vi "mp285.vi"() -> ()   [LabVIEW 2018]
uses:
  <vilib>/Instr/_visa.llb/VISA Configure Serial Port (Instr).vi
panel:
  out "Z.":dbl
  out "Y.":dbl
  out "X.":dbl
  in  "获取当前位置":bool
  out "字符串":string
  in  "VISA资源名称":refnum<visa-resource-name>
  in  "设置精度和速度":bool
  in  "获取当前速度和位置":bool
  in  "相对运动":bool
  in  "绝对运动":bool
  in  "重置":bool
  in  "中断移动":bool
  in  "设置当前位置为原点":bool
  in  "停止":bool
  out "速度":dbl
  out "精度":u16
  in  "速度":dbl
  in  "精度":u16(ring)=10 items=["Low (10microsteps/step)", "High (50microsteps/step)"]
  out "错误输出":errorcluster
  in  "Abso_Z":dbl
  in  "Abso_Y":dbl
  in  "Abso_X":dbl
  in  "Z":dbl
  in  "Y":dbl
  in  "X":dbl
  in  "停止位 (10: 1位)":u16(ring)=10 caption="停止位(1)" items=["1.0"=10, "1.5"=15, "2.0"=20]
  in  "校验（无）":enum16{"None", "Odd", "Even", "Mark", "Space"}(ring)
  in  "波特率(9600)":u32=9600
  # "当前位置\n（单位：微米）"
  # "移动到绝对位置\n（单位：微米）"
  # "移动到相对位置\n（单位：微米）"
  # "串口设置"
  # "获取精度和速度"
  # "设置精度和速度"
  # "速度范围：低精度模式下0-3000微米/秒\n               高精度模式下0-1310微米/秒"
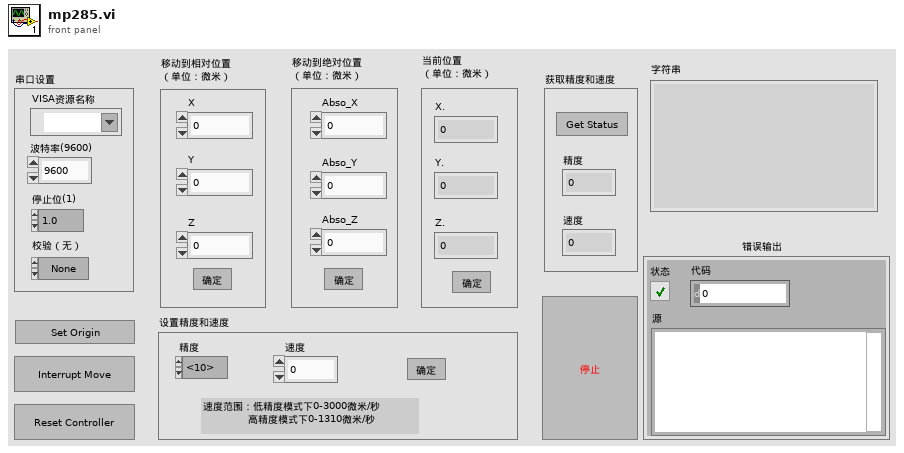
[diagram p1: front panel]
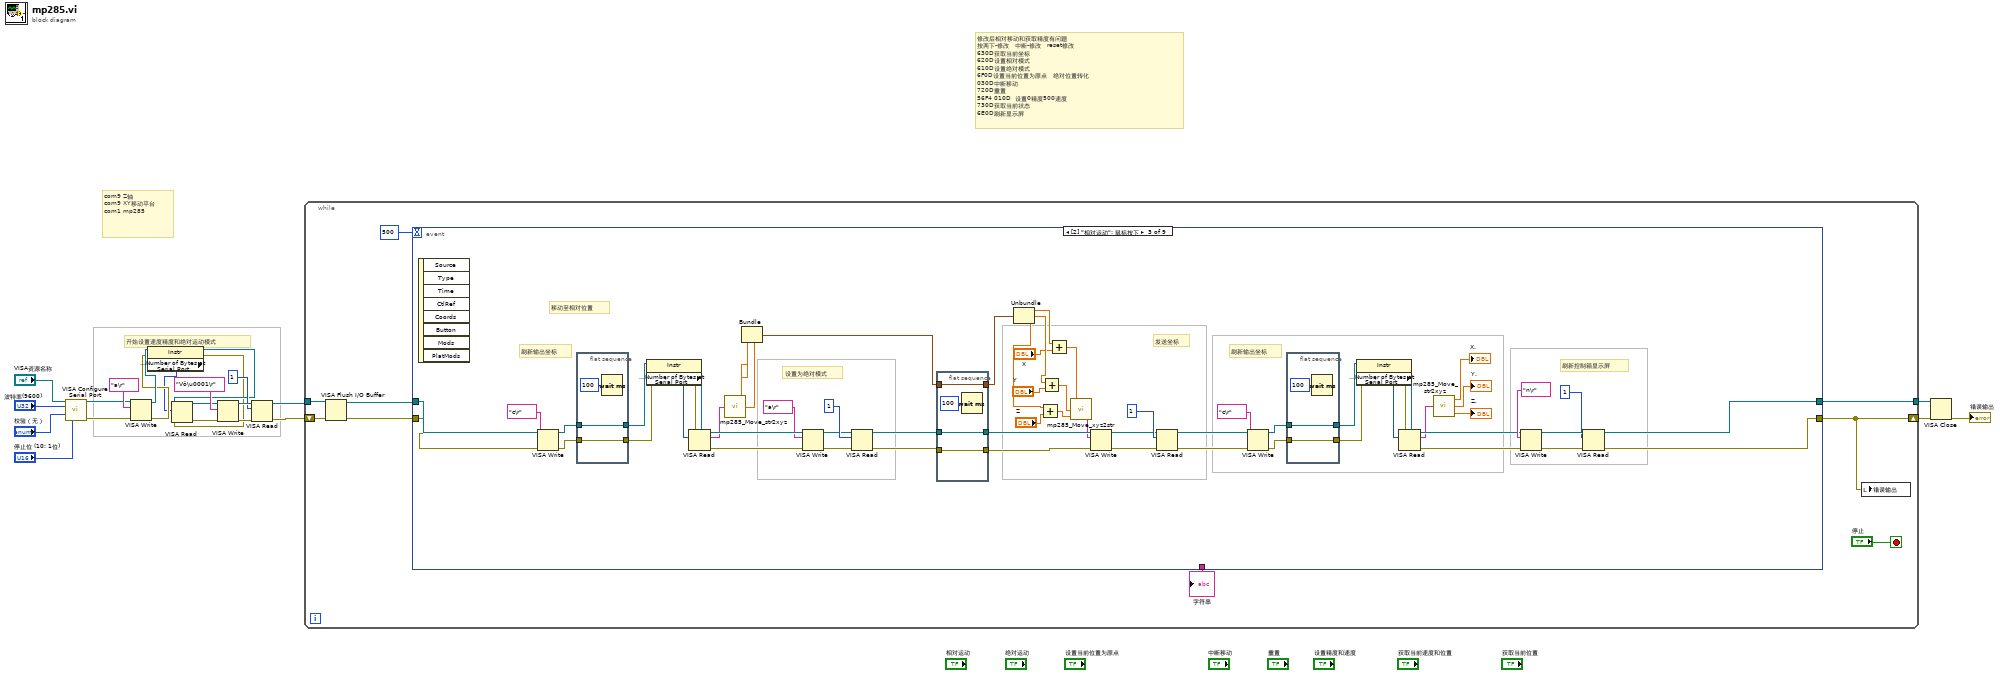
[diagram p0: block diagram]
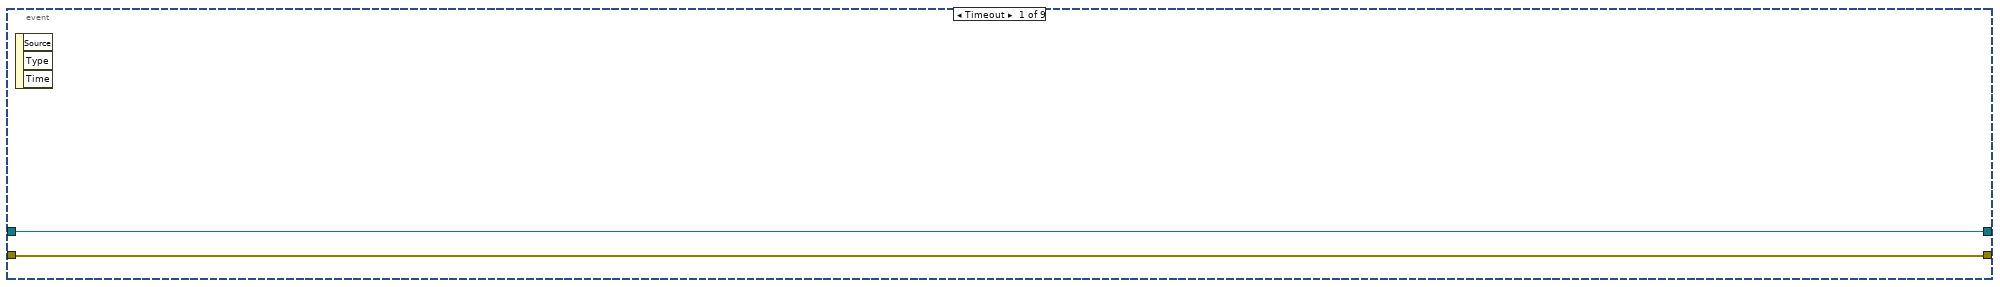
[diagram p2: hidden frame]
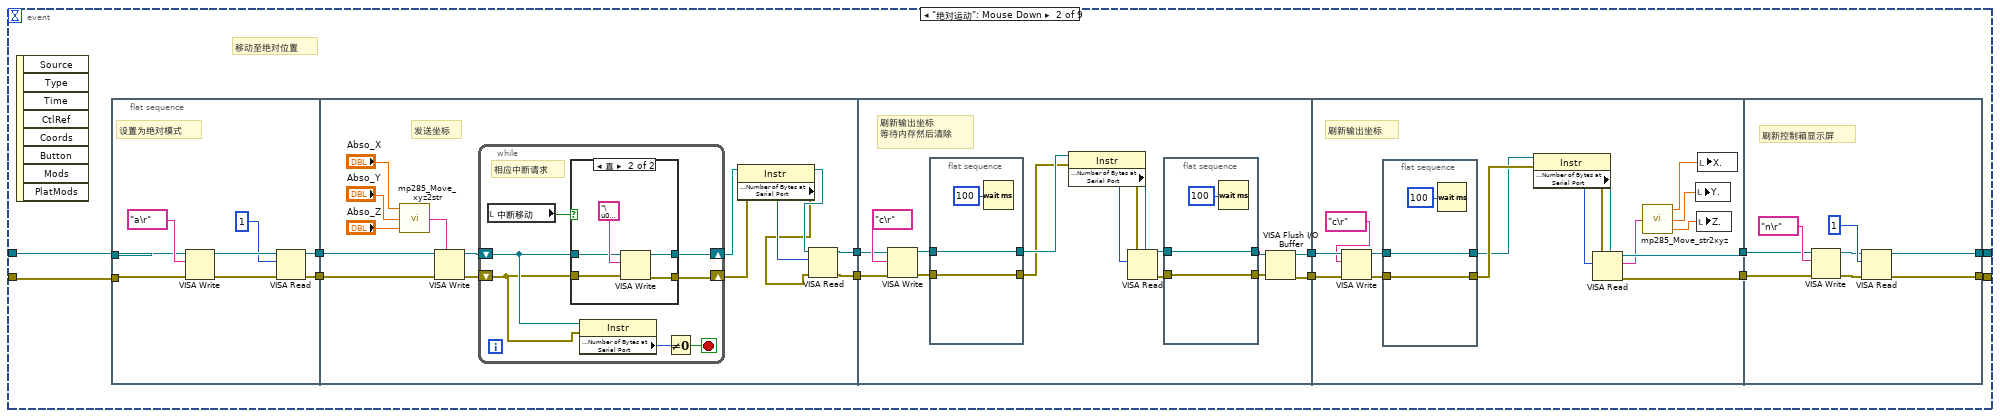
[diagram p3: hidden frame]
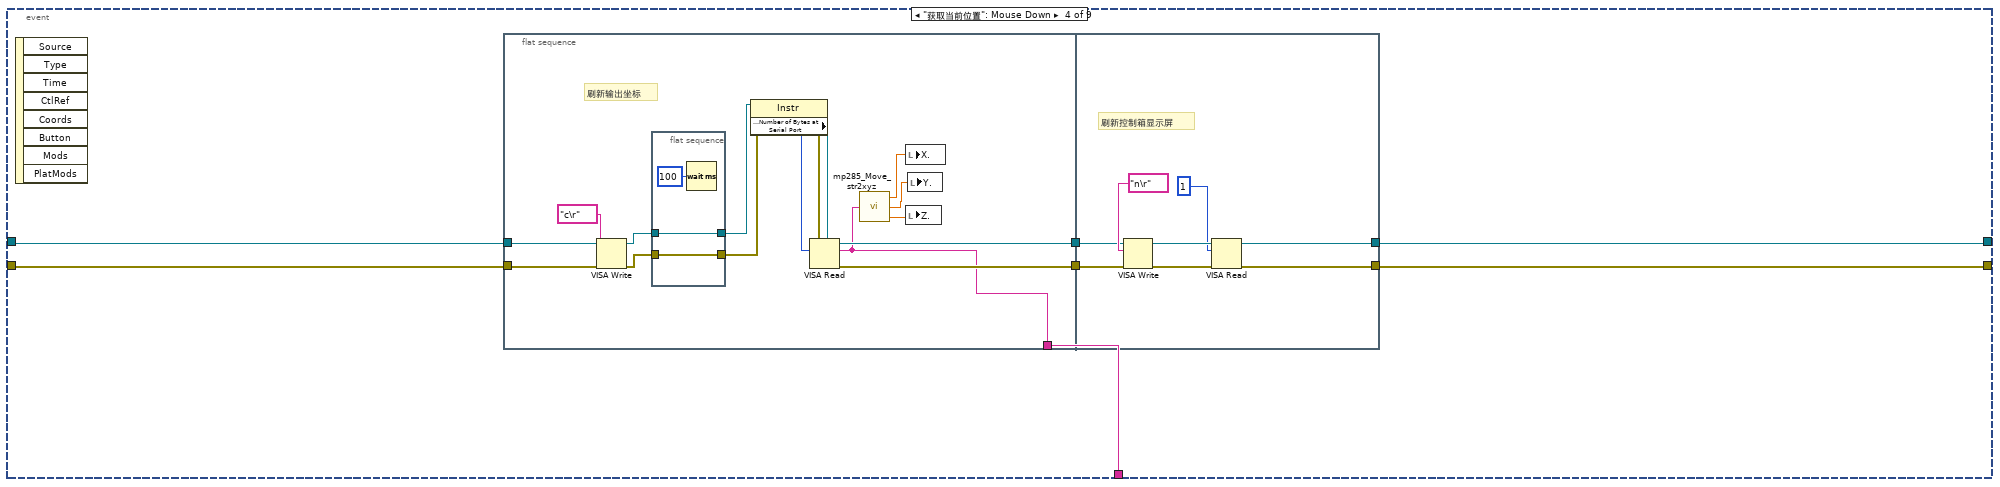
[diagram p5: hidden frame]
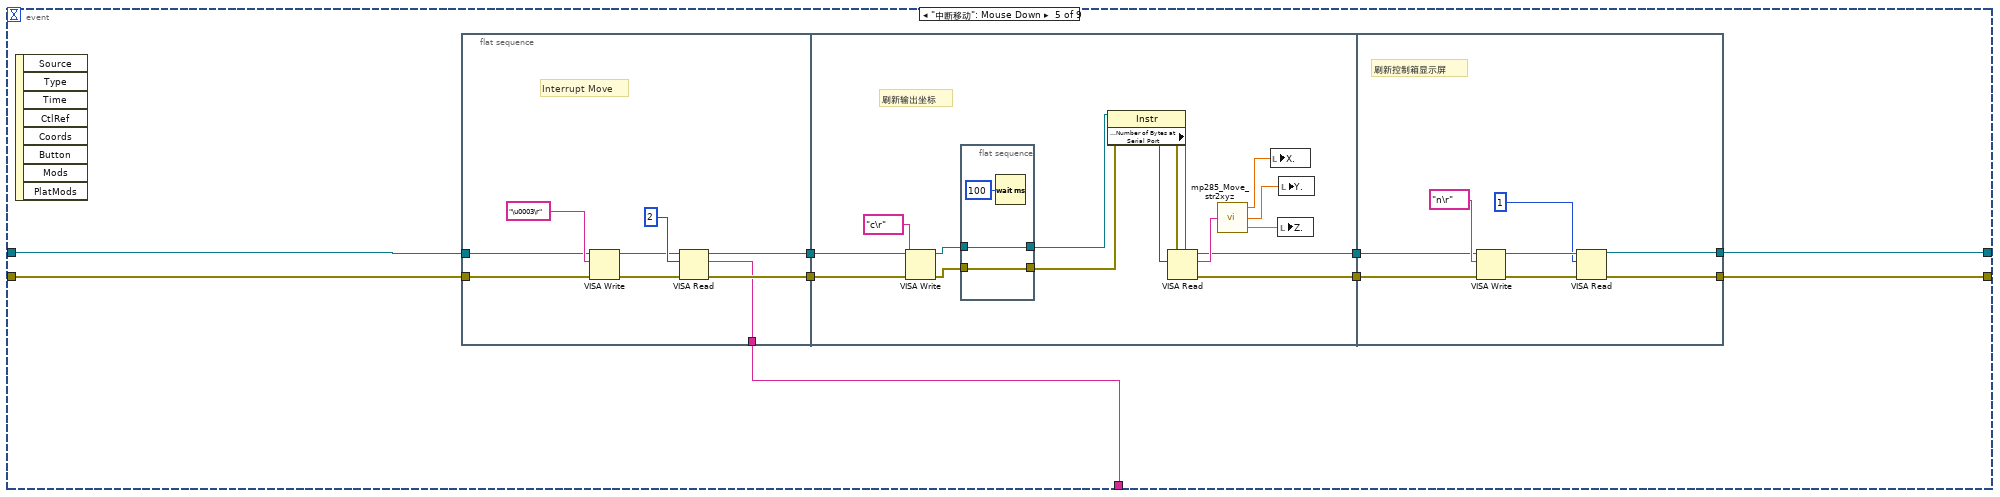
[diagram p6: hidden frame]
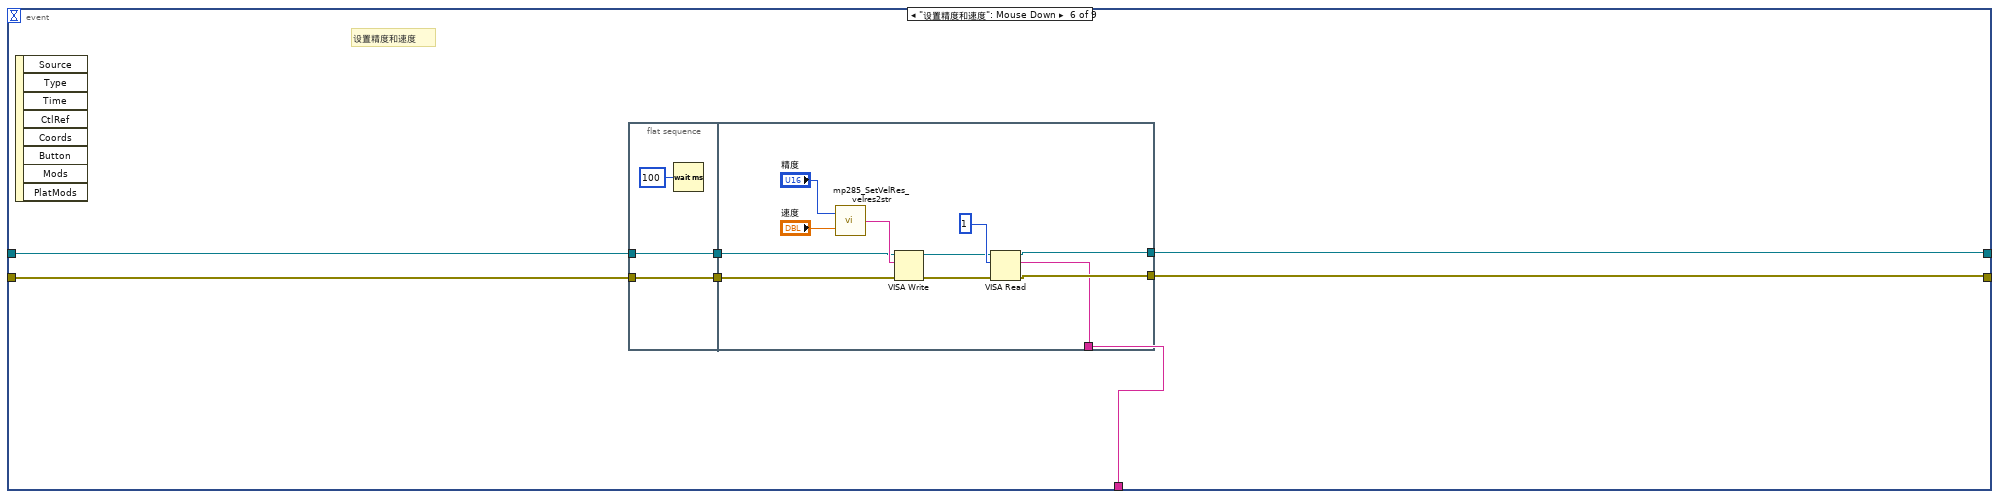
[diagram p7: hidden frame]
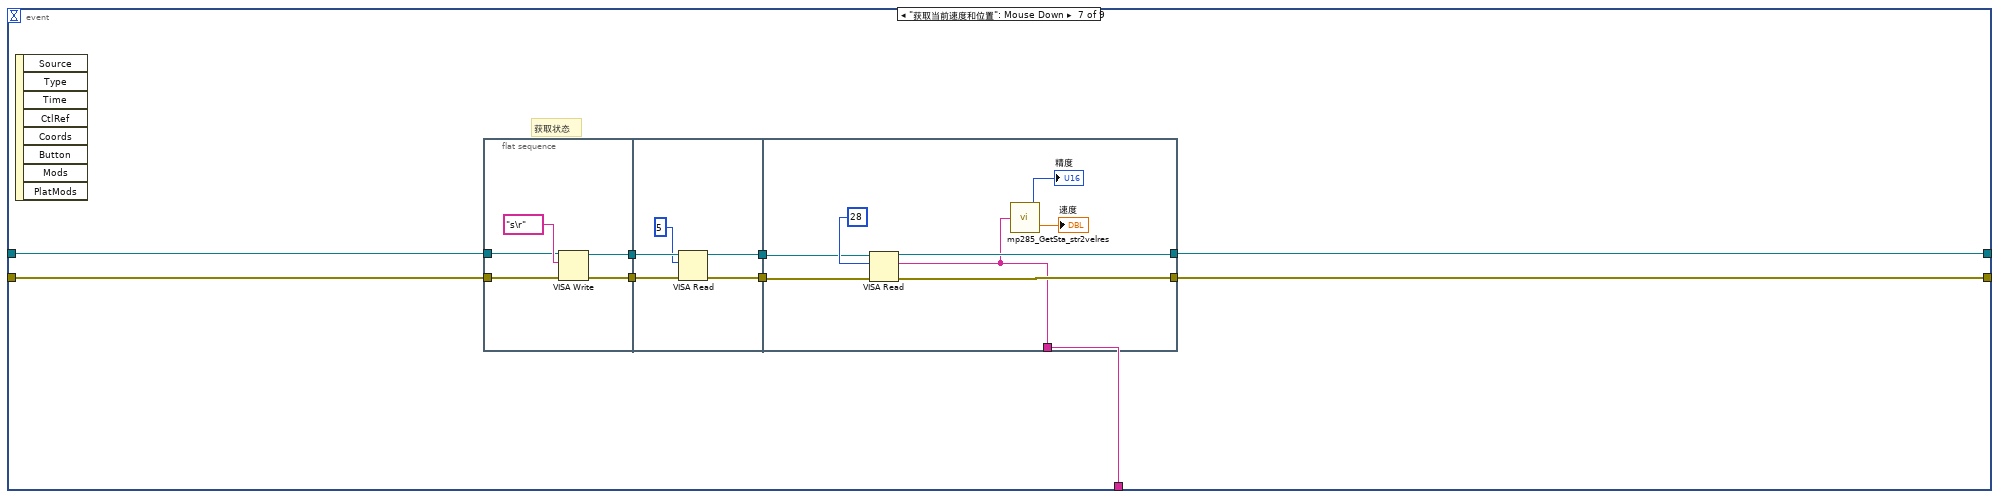
[diagram p8: hidden frame]
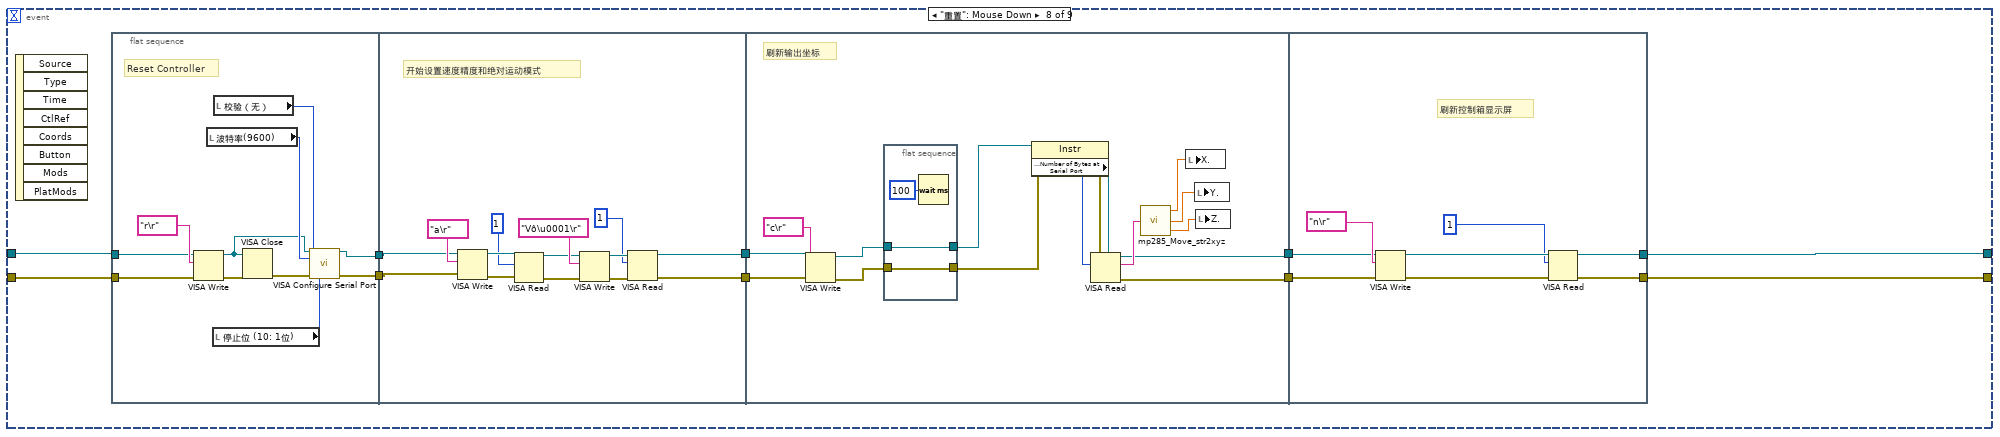
[diagram p9: hidden frame]
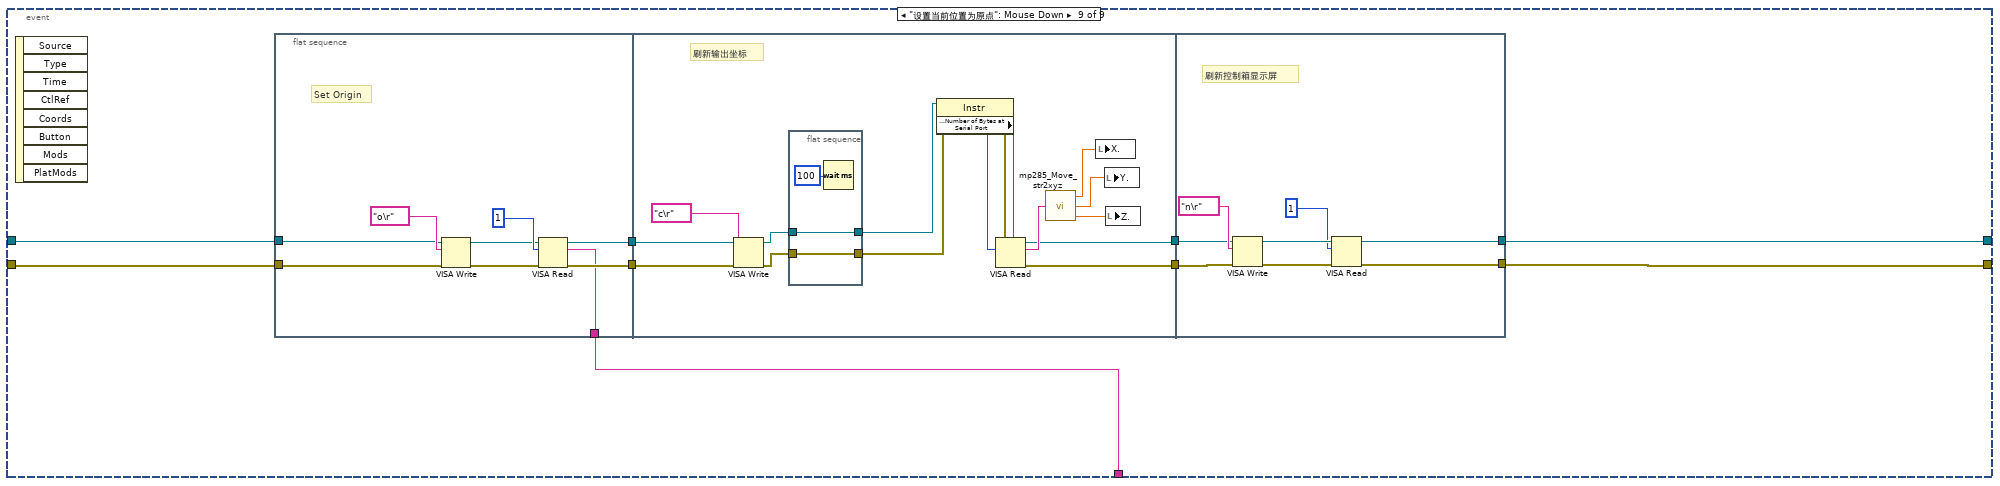
[diagram p10: hidden frame]
diagram:
  # "com9 Z轴\ncom9 XY移动平台\ncom1 mp285"
  # "开始设置速度精度和绝对运动模式"
  # "修改后相对移动和获取精度有问题\n按两下-修改   中断-修改   reset修改\n630D获取当前坐标\n620D设置相对模式\n610D设置绝对模式\n6F0D设置当前位置为原点   绝对位置转化\n030D中断移动\n720D重置\n56F4 010D  设置0精度500速度\n730D获取当前状态\n6E0D刷新显示屏"
  n1 = call-poly "VISA Configure Serial Port"("VISA resource name"="VISA资源名称", "baud rate (9600)"="波特率(9600)", "parity (0:none)"="校验（无）", "stop bits (10: 1 bit)"="停止位 (10: 1位)") -> ("VISA resource name out"=w7:refnum<visa-resource-name>, "error out"=w6:errorcluster)  [unwired: 10 in]
  n2 = VISA Write ("VISA写入")(VISA resource name=w7, write buffer="a\r" ("写入缓冲区"), error in (no error)=w6) -> (VISA resource name out=w5:refnum<visa-resource-name>, error out=w4:errorcluster)  [unwired: 1 out]
  n3 = property class="Instr"(reference=w5, error in=w4) -> (reference out=w3:refnum<visa-resource-name>, error out=w1:errorcluster, "Serial Settings:Number of Bytes at Serial Port"=w2:u32)
  n4 = VISA Read(VISA resource name=w3, byte count=w2, error in (no error)=w1) -> (VISA resource name out=w14:refnum<visa-resource-name>, error out=w13:errorcluster)  [unwired: 2 out]
  n5 = VISA Write ("VISA写入")(VISA resource name=w14, write buffer="Vô\u0001\r" ("写入缓冲区"), error in (no error)=w13) -> (VISA resource name out=w11:refnum<visa-resource-name>, error out=w12:errorcluster)  [unwired: 1 out]
  n6 = VISA Read(VISA resource name=w11, byte count=u32 1 ("字节总数"), error in (no error)=w12) -> (VISA resource name out=w10:refnum<visa-resource-name>, error out=w8:errorcluster)  [unwired: 2 out]
  n7 = while {
    tunnel: w10 -> [w27]
    tunnel: [w31] -> w18
    shift-right: [w28] -> w17
    shift-left: w8 -> [w25]
    stop <- "停止" stop-if-true
    n8 = VISA Flush I/O Buffer(VISA resource name=w27, error in (no error)=w25) -> (VISA resource name out=w26:refnum<visa-resource-name>, error out=w24:errorcluster)  [unwired: 1 in]
    n9 = event shown="[2] \"相对运动\": 鼠标按下" {
      selector: _ -> [_ _ _ _ _ _ _ _ _]
      dyn-events: _ -> [_ _ _ _ _ _ _ _ _]
      timeout: 500 -> [_ _ _ _ _ _ _ _ _]
      tunnel: w26 -> [w34 w46 w143 w210 w245 w289 w305 w340 w401]
      tunnel: w24 -> [w33 w45 w142 w209 w246 w288 w304 w339 w400]
      tunnel: [w33 w39 w137 w204 w238 w286 w307 w331 w393] -> w28
      tunnel: [w34 w40 w138 w205 w239 w287 w308 w332 w394] -> w31
      tunnel: [_ _ _ w208 w244 w285 w306 _ w399] -> w30
      event Timeout {
        n10 = event-data() -> ()  [unwired: 1 in, 3 out]
      }
      event "绝对运动": Mouse Down {
        # "移动至绝对位置"
        n11 = event-data() -> ()  [unwired: 1 in, 8 out]
        n12 = flat-sequence {
          tunnel: w46 -> [w50]
          tunnel: w45 -> [w49]
          tunnel: [w48] -> w44
          tunnel: [w47] -> w43
          tunnel: w44 -> [w59]
          tunnel: w43 -> [w58]
          tunnel: [w57] -> w42
          tunnel: [w56] -> w41
          tunnel: w42 -> [w95]
          tunnel: w41 -> [w94]
          tunnel: [w88] -> w38
          tunnel: [w89] -> w37
          tunnel: w38 -> [w114]
          tunnel: w37 -> [w113]
          tunnel: [w111] -> w36
          tunnel: [w110] -> w35
          tunnel: [w129] -> w40
          tunnel: [w128] -> w39
          tunnel: w36 -> [w126]
          tunnel: w35 -> [w125]
          frame #0 {
            # "设置为绝对模式"
            n13 = VISA Write ("VISA写入")(VISA resource name=w50, write buffer="a\r" ("写入缓冲区"), error in (no error)=w49) -> (VISA resource name out=w53:refnum<visa-resource-name>, error out=w52:errorcluster)  [unwired: 1 out]
            n14 = VISA Read(VISA resource name=w53, byte count=u32 1 ("字节总数"), error in (no error)=w52) -> (VISA resource name out=w47:refnum<visa-resource-name>, error out=w48:errorcluster)  [unwired: 2 out]
          }
          frame #1 {
            # "发送坐标"
            n15 = call "mp285_Move_xyz2str.vi"("Z轴"="Abso_Z", "Y轴"="Abso_Y", "X轴"="Abso_X") -> ("发送至串口的字符串"=w69:string)
            n16 = VISA Write ("VISA写入")(VISA resource name=w58, write buffer=w69, error in (no error)=w59) -> (VISA resource name out=w65:refnum<visa-resource-name>, error out=w64:errorcluster)  [unwired: 1 out]
            n17 = while {
              shift-right: [w75] -> w63
              shift-left: w65 -> [w73]
              shift-right: [w74] -> w62
              shift-left: w64 -> [w72]
              stop <- w71 stop-if-true
              # "相应中断请求"
              n18 = local read "中断移动"() -> (w76:bool)
              n19 = case shown="真" w76 {
                tunnel: [w77 w80] -> w75
                tunnel: [w78 w79] -> w74
                tunnel: w73 -> [w77 w82]
                tunnel: w72 -> [w78 w81]
                frame False {
                }
                frame True {
                  n20 = VISA Write ("VISA写入")(VISA resource name=w82, write buffer="\u0003" ("写入缓冲区"), error in (no error)=w81) -> (VISA resource name out=w80:refnum<visa-resource-name>, error out=w79:errorcluster)  [unwired: 1 out]
                }
              }
              n21 = property class="Instr"(reference=w73, error in=w72) -> ("Serial Settings:Number of Bytes at Serial Port"=w70:u32)  [unwired: 2 out]
              n22 = Not Equal To 0?(x=w70) -> (x != 0?=w71:bool)
            }
            n23 = property class="Instr"(reference=w63, error in=w62) -> (reference out=w61:refnum<visa-resource-name>, error out=w55:errorcluster, "Serial Settings:Number of Bytes at Serial Port"=w60:u32)
            n24 = VISA Read(VISA resource name=w61, byte count=w60, error in (no error)=w55) -> (VISA resource name out=w57:refnum<visa-resource-name>, error out=w56:errorcluster)  [unwired: 2 out]
          }
          frame #2 {
            # "刷新输出坐标\n等待内存然后清除"
            n25 = VISA Write ("VISA写入")(VISA resource name=w95, write buffer="c\r" ("写入缓冲区"), error in (no error)=w94) -> (VISA resource name out=w93:refnum<visa-resource-name>, error out=w92:errorcluster)  [unwired: 1 out]
            n26 = flat-sequence {
              tunnel: w93 -> [w104]
              tunnel: w92 -> [w103]
              tunnel: [w104] -> w91
              tunnel: [w103] -> w90
              frame #0 {
                n27 = Wait (ms)(milliseconds to wait=u32 100 ("等待时间（毫秒）")) -> ()  [unwired: 1 out]
              }
            }
            n28 = property class="Instr"(reference=w91, error in=w90) -> (reference out=w98:refnum<visa-resource-name>, error out=w99:errorcluster, "Serial Settings:Number of Bytes at Serial Port"=w97:u32)
            n29 = VISA Read(VISA resource name=w98, byte count=w97, error in (no error)=w99) -> (VISA resource name out=w87:refnum<visa-resource-name>, error out=w86:errorcluster)  [unwired: 2 out]
            n30 = flat-sequence {
              tunnel: w87 -> [w101]
              tunnel: w86 -> [w100]
              tunnel: [w101] -> w85
              tunnel: [w100] -> w84
              frame #0 {
                n31 = Wait (ms)(milliseconds to wait=u32 100 ("等待时间（毫秒）")) -> ()  [unwired: 1 out]
              }
            }
            n32 = VISA Flush I/O Buffer(VISA resource name=w85, error in (no error)=w84) -> (VISA resource name out=w88:refnum<visa-resource-name>, error out=w89:errorcluster)  [unwired: 1 in]
          }
          frame #3 {
            # "刷新输出坐标"
            n33 = VISA Write ("VISA写入")(VISA resource name=w114, write buffer="c\r" ("写入缓冲区"), error in (no error)=w113) -> (VISA resource name out=w118:refnum<visa-resource-name>, error out=w119:errorcluster)  [unwired: 1 out]
            n34 = flat-sequence {
              tunnel: w118 -> [w123]
              tunnel: w119 -> [w122]
              tunnel: [w123] -> w120
              tunnel: [w122] -> w121
              frame #0 {
                n35 = Wait (ms)(milliseconds to wait=u32 100 ("等待时间（毫秒）")) -> ()  [unwired: 1 out]
              }
            }
            n36 = property class="Instr"(reference=w120, error in=w121) -> (reference out=w116:refnum<visa-resource-name>, error out=w115:errorcluster, "Serial Settings:Number of Bytes at Serial Port"=w117:u32)
            n37 = VISA Read(VISA resource name=w116, byte count=w117, error in (no error)=w115) -> (VISA resource name out=w111:refnum<visa-resource-name>, read buffer=w109:string, error out=w110:errorcluster)  [unwired: 1 out]
            n38 = call "mp285_Move_str2xyz.vi"("字符串"=w109) -> ("X轴"=w108:dbl, "Y轴"=w107:dbl, "Z轴"=w106:dbl)
            n39 = local write "Y."(w107) -> ()
            n40 = local write "Z."(w106) -> ()
            n41 = local write "X."(w108) -> ()
          }
          frame #4 {
            # "刷新控制箱显示屏"
            n42 = VISA Write ("VISA写入")(VISA resource name=w126, write buffer="n\r" ("写入缓冲区"), error in (no error)=w125) -> (VISA resource name out=w131:refnum<visa-resource-name>, error out=w130:errorcluster)  [unwired: 1 out]
            n43 = VISA Read(VISA resource name=w131, byte count=u32 1 ("字节总数"), error in (no error)=w130) -> (VISA resource name out=w129:refnum<visa-resource-name>, error out=w128:errorcluster)  [unwired: 2 out]
          }
        }
      }
      event "相对运动": Mouse Down {
        # "刷新输出坐标"
        # "刷新输出坐标"
        # "刷新控制箱显示屏"
        # "设置为绝对模式"
        # "发送坐标"
        # "移动至相对位置"
        n44 = event-data() -> ()  [unwired: 1 in, 8 out]
        n45 = VISA Write ("VISA写入")(VISA resource name=w143, write buffer="c\r" ("写入缓冲区"), error in (no error)=w142) -> (VISA resource name out=w171:refnum<visa-resource-name>, error out=w170:errorcluster)  [unwired: 1 out]
        n46 = flat-sequence {
          tunnel: [w199] -> w168
          tunnel: w171 -> [w199]
          tunnel: [w198] -> w169
          tunnel: w170 -> [w198]
          frame #0 {
            n47 = Wait (ms)(milliseconds to wait=u32 100 ("等待时间（毫秒）")) -> ()  [unwired: 1 out]
          }
        }
        n48 = property class="Instr"(reference=w168, error in=w169) -> (reference out=w173:refnum<visa-resource-name>, error out=w172:errorcluster, "Serial Settings:Number of Bytes at Serial Port"=w174:u32)
        n49 = VISA Read(VISA resource name=w173, byte count=w174, error in (no error)=w172) -> (VISA resource name out=w180:refnum<visa-resource-name>, read buffer=w176:string, error out=w181:errorcluster)  [unwired: 1 out]
        n50 = call "mp285_Move_str2xyz.vi"("字符串"=w176) -> ("X轴"=w184:dbl, "Y轴"=w185:dbl, "Z轴"=w186:dbl)
        n51 = Bundle("X轴"=w184, "Y轴"=w185, "Z轴"=w186) -> (w189:cluster{"X轴":dbl, "Y轴":dbl, "Z轴":dbl})  [unwired: 1 in]
        n52 = VISA Write ("VISA写入")(VISA resource name=w180, write buffer="a\r" ("写入缓冲区"), error in (no error)=w181) -> (VISA resource name out=w144:refnum<visa-resource-name>, error out=w145:errorcluster)  [unwired: 1 out]
        n53 = VISA Read(VISA resource name=w144, byte count=u32 1 ("字节总数"), error in (no error)=w145) -> (VISA resource name out=w187:refnum<visa-resource-name>, error out=w188:errorcluster)  [unwired: 2 out]
        n54 = flat-sequence {
          tunnel: w187 -> [w196]
          tunnel: w188 -> [w195]
          tunnel: [w196] -> w182
          tunnel: [w195] -> w183
          tunnel: w189 -> [w194]
          tunnel: [w194] -> w190
          frame #0 {
            n55 = Wait (ms)(milliseconds to wait=u32 100 ("等待时间（毫秒）")) -> ()  [unwired: 1 out]
          }
        }
        n56 = Unbundle(w190) -> ("X轴"=w191:dbl, "Y轴"=w192:dbl, "Z轴"=w193:dbl)
        n57 = Add(x=w193, y="Z") -> (x+y=w177:dbl)
        n58 = Add(x=w192, y="Y") -> (x+y=w178:dbl)
        n59 = Add(x=w191, y="X") -> (x+y=w179:dbl)
        n60 = call "mp285_Move_xyz2str.vi"("Z轴"=w177, "Y轴"=w178, "X轴"=w179) -> ("发送至串口的字符串"=w150:string)
        n61 = VISA Write ("VISA写入")(VISA resource name=w182, write buffer=w150, error in (no error)=w183) -> (VISA resource name out=w148:refnum<visa-resource-name>, error out=w147:errorcluster)  [unwired: 1 out]
        n62 = VISA Read(VISA resource name=w148, byte count=u32 1 ("字节总数"), error in (no error)=w147) -> (VISA resource name out=w166:refnum<visa-resource-name>, error out=w167:errorcluster)  [unwired: 2 out]
        n63 = VISA Write ("VISA写入")(VISA resource name=w166, write buffer="c\r" ("写入缓冲区"), error in (no error)=w167) -> (VISA resource name out=w155:refnum<visa-resource-name>, error out=w154:errorcluster)  [unwired: 1 out]
        n64 = flat-sequence {
          tunnel: [w202] -> w152
          tunnel: w155 -> [w202]
          tunnel: [w201] -> w153
          tunnel: w154 -> [w201]
          frame #0 {
            n65 = Wait (ms)(milliseconds to wait=u32 100 ("等待时间（毫秒）")) -> ()  [unwired: 1 out]
          }
        }
        n66 = property class="Instr"(reference=w152, error in=w153) -> (reference out=w157:refnum<visa-resource-name>, error out=w156:errorcluster, "Serial Settings:Number of Bytes at Serial Port"=w158:u32)
        n67 = VISA Read(VISA resource name=w157, byte count=w158, error in (no error)=w156) -> (VISA resource name out=w160:refnum<visa-resource-name>, read buffer=w136:string, error out=w159:errorcluster)  [unwired: 1 out]
        n68 = call "mp285_Move_str2xyz.vi"("字符串"=w136) -> ("X轴"=→"X.":dbl, "Y轴"=→"Y.":dbl, "Z轴"=→"Z.":dbl)
        n69 = VISA Write ("VISA写入")(VISA resource name=w160, write buffer="n\r" ("写入缓冲区"), error in (no error)=w159) -> (VISA resource name out=w164:refnum<visa-resource-name>, error out=w165:errorcluster)  [unwired: 1 out]
        n70 = VISA Read(VISA resource name=w164, byte count=u32 1 ("字节总数"), error in (no error)=w165) -> (VISA resource name out=w138:refnum<visa-resource-name>, error out=w137:errorcluster)  [unwired: 2 out]
      }
      event "获取当前位置": Mouse Down {
        n71 = event-data() -> ()  [unwired: 1 in, 8 out]
        n72 = flat-sequence {
          tunnel: w210 -> [w216]
          tunnel: w209 -> [w215]
          tunnel: [w214] -> w208
          tunnel: [w219] -> w207
          tunnel: [w218] -> w206
          tunnel: w207 -> [w232]
          tunnel: w206 -> [w233]
          tunnel: [w231] -> w205
          tunnel: [w230] -> w204
          frame #0 {
            # "刷新输出坐标"
            n73 = VISA Write ("VISA写入")(VISA resource name=w216, write buffer="c\r" ("写入缓冲区"), error in (no error)=w215) -> (VISA resource name out=w223:refnum<visa-resource-name>, error out=w224:errorcluster)  [unwired: 1 out]
            n74 = flat-sequence {
              tunnel: [w228] -> w226
              tunnel: w223 -> [w228]
              tunnel: [w227] -> w225
              tunnel: w224 -> [w227]
              frame #0 {
                n75 = Wait (ms)(milliseconds to wait=u32 100 ("等待时间（毫秒）")) -> ()  [unwired: 1 out]
              }
            }
            n76 = property class="Instr"(reference=w226, error in=w225) -> (reference out=w221:refnum<visa-resource-name>, error out=w222:errorcluster, "Serial Settings:Number of Bytes at Serial Port"=w220:u32)
            n77 = VISA Read(VISA resource name=w221, byte count=w220, error in (no error)=w222) -> (VISA resource name out=w218:refnum<visa-resource-name>, read buffer=w214:string, error out=w219:errorcluster)  [unwired: 1 out]
            n78 = call "mp285_Move_str2xyz.vi"("字符串"=w214) -> ("X轴"=w213:dbl, "Y轴"=w212:dbl, "Z轴"=w211:dbl)
            n79 = local write "X."(w213) -> ()
            n80 = local write "Z."(w211) -> ()
            n81 = local write "Y."(w212) -> ()
          }
          frame #1 {
            # "刷新控制箱显示屏"
            n82 = VISA Write ("VISA写入")(VISA resource name=w233, write buffer="n\r" ("写入缓冲区"), error in (no error)=w232) -> (VISA resource name out=w236:refnum<visa-resource-name>, error out=w237:errorcluster)  [unwired: 1 out]
            n83 = VISA Read(VISA resource name=w236, byte count=u32 1 ("字节总数"), error in (no error)=w237) -> (VISA resource name out=w231:refnum<visa-resource-name>, error out=w230:errorcluster)  [unwired: 2 out]
          }
        }
      }
      event "中断移动": Mouse Down {
        n84 = event-data() -> ()  [unwired: 1 in, 8 out]
        n85 = flat-sequence {
          tunnel: w246 -> [w252]
          tunnel: w245 -> [w251]
          tunnel: [w247] -> w244
          tunnel: [w249] -> w243
          tunnel: [w248] -> w242
          tunnel: w243 -> [w262]
          tunnel: w242 -> [w261]
          tunnel: [w260] -> w241
          tunnel: [w259] -> w240
          tunnel: w241 -> [w278]
          tunnel: w240 -> [w277]
          tunnel: [w276] -> w239
          tunnel: [w275] -> w238
          frame #0 {
            # "Interrupt Move"
            n86 = VISA Write ("VISA写入")(VISA resource name=w251, write buffer="\u0003\r" ("写入缓冲区"), error in (no error)=w252) -> (VISA resource name out=w250:refnum<visa-resource-name>, error out=w253:errorcluster)  [unwired: 1 out]
            n87 = VISA Read(VISA resource name=w250, byte count=u32 2 ("字节总数"), error in (no error)=w253) -> (VISA resource name out=w249:refnum<visa-resource-name>, read buffer=w247:string, error out=w248:errorcluster)  [unwired: 1 out]
          }
          frame #1 {
            # "刷新输出坐标"
            n88 = VISA Write ("VISA写入")(VISA resource name=w262, write buffer="c\r" ("写入缓冲区"), error in (no error)=w261) -> (VISA resource name out=w266:refnum<visa-resource-name>, error out=w265:errorcluster)  [unwired: 1 out]
            n89 = flat-sequence {
              tunnel: [w273] -> w263
              tunnel: w266 -> [w273]
              tunnel: [w272] -> w264
              tunnel: w265 -> [w272]
              frame #0 {
                n90 = Wait (ms)(milliseconds to wait=u32 100 ("等待时间（毫秒）")) -> ()  [unwired: 1 out]
              }
            }
            n91 = property class="Instr"(reference=w263, error in=w264) -> (reference out=w268:refnum<visa-resource-name>, error out=w267:errorcluster, "Serial Settings:Number of Bytes at Serial Port"=w269:u32)
            n92 = VISA Read(VISA resource name=w268, byte count=w269, error in (no error)=w267) -> (VISA resource name out=w260:refnum<visa-resource-name>, read buffer=w271:string, error out=w259:errorcluster)  [unwired: 1 out]
            n93 = call "mp285_Move_str2xyz.vi"("字符串"=w271) -> ("X轴"=w258:dbl, "Y轴"=w257:dbl, "Z轴"=w256:dbl)
            n94 = local write "X."(w258) -> ()
            n95 = local write "Z."(w256) -> ()
            n96 = local write "Y."(w257) -> ()
          }
          frame #2 {
            # "刷新控制箱显示屏"
            n97 = VISA Write ("VISA写入")(VISA resource name=w278, write buffer="n\r" ("写入缓冲区"), error in (no error)=w277) -> (VISA resource name out=w281:refnum<visa-resource-name>, error out=w282:errorcluster)  [unwired: 1 out]
            n98 = VISA Read(VISA resource name=w281, byte count=u32 1 ("字节总数"), error in (no error)=w282) -> (VISA resource name out=w276:refnum<visa-resource-name>, error out=w275:errorcluster)  [unwired: 2 out]
          }
        }
      }
      event "设置精度和速度": Mouse Down {
        # "设置精度和速度"
        n99 = event-data() -> ()  [unwired: 1 in, 8 out]
        n100 = flat-sequence {
          tunnel: w288 -> [w291]
          tunnel: w289 -> [w292]
          tunnel: [w292] -> w284
          tunnel: [w291] -> w283
          tunnel: [w295] -> w287
          tunnel: [w294] -> w286
          tunnel: [w293] -> w285
          tunnel: w284 -> [w299]
          tunnel: w283 -> [w298]
          frame #0 {
            n101 = Wait (ms)(milliseconds to wait=u32 100 ("等待时间（毫秒）")) -> ()  [unwired: 1 out]
          }
          frame #1 {
            n102 = call "mp285_SetVelRes_velres2str.vi"("速度"="速度", "精度"="精度") -> ("发送至串口的字符串"=w300:string)
            n103 = VISA Write ("VISA写入")(VISA resource name=w299, write buffer=w300, error in (no error)=w298) -> (VISA resource name out=w302:refnum<visa-resource-name>, error out=w301:errorcluster)  [unwired: 1 out]
            n104 = VISA Read(VISA resource name=w302, byte count=u32 1 ("字节总数"), error in (no error)=w301) -> (VISA resource name out=w295:refnum<visa-resource-name>, read buffer=w293:string, error out=w294:errorcluster)  [unwired: 1 out]
          }
        }
      }
      event "获取当前速度和位置": Mouse Down {
        # "获取状态"
        n105 = event-data() -> ()  [unwired: 1 in, 8 out]
        n106 = flat-sequence {
          tunnel: w305 -> [w314]
          tunnel: w304 -> [w313]
          tunnel: [w316] -> w312
          tunnel: [w315] -> w311
          tunnel: w312 -> [w322]
          tunnel: w311 -> [w319]
          tunnel: [w321] -> w310
          tunnel: [w320] -> w309
          tunnel: w310 -> [w327]
          tunnel: w309 -> [w326]
          tunnel: [w325] -> w308
          tunnel: [w324] -> w307
          tunnel: [w323] -> w306
          frame #0 {
            n107 = VISA Write ("VISA写入")(VISA resource name=w314, write buffer="s\r" ("写入缓冲区"), error in (no error)=w313) -> (VISA resource name out=w316:refnum<visa-resource-name>, error out=w315:errorcluster)  [unwired: 1 out]
          }
          frame #1 {
            n108 = VISA Read(VISA resource name=w322, byte count=u32 5 ("字节总数"), error in (no error)=w319) -> (VISA resource name out=w321:refnum<visa-resource-name>, error out=w320:errorcluster)  [unwired: 2 out]
          }
          frame #2 {
            n109 = VISA Read(VISA resource name=w327, byte count=u32 28 ("字节总数"), error in (no error)=w326) -> (VISA resource name out=w325:refnum<visa-resource-name>, read buffer=w323:string, error out=w324:errorcluster)  [unwired: 1 out]
            n110 = call "mp285_GetSta_str2velres.vi"("字符串"=w323) -> ("精度"=→"精度":u16, "速度"=→"速度":dbl)
          }
        }
      }
      event "重置": Mouse Down {
        n111 = event-data() -> ()  [unwired: 1 in, 8 out]
        n112 = flat-sequence {
          tunnel: w340 -> [w350]
          tunnel: w339 -> [w349]
          tunnel: [w343] -> w338
          tunnel: [w342] -> w337
          tunnel: w338 -> [w355]
          tunnel: w337 -> [w354]
          tunnel: [w353] -> w336
          tunnel: [w352] -> w335
          tunnel: w336 -> [w372]
          tunnel: w335 -> [w371]
          tunnel: [w370] -> w334
          tunnel: [w369] -> w333
          tunnel: w334 -> [w388]
          tunnel: w333 -> [w387]
          tunnel: [w386] -> w332
          tunnel: [w385] -> w331
          frame #0 {
            # "Reset Controller"
            n113 = VISA Write ("VISA写入")(VISA resource name=w350, write buffer="r\r" ("写入缓冲区"), error in (no error)=w349) -> (VISA resource name out=w341:refnum<visa-resource-name>, error out=w348:errorcluster)  [unwired: 1 out]
            n114 = local read "波特率(9600)"() -> (w346:u32)
            n115 = local read "停止位 (10: 1位)"() -> (w344:u16)
            n116 = local read "校验（无）"() -> (w345:enum16{"None", "Odd", "Even", "Mark", "Space"})
            n117 = VISA Close(VISA resource name=w341, error in (no error)=w348) -> (error out=w347:errorcluster)
            n118 = call-poly "VISA Configure Serial Port"("VISA resource name"=w341, "baud rate (9600)"=w346, "parity (0:none)"=w345, "error in (no error)"=w347, "stop bits (10: 1 bit)"=w344) -> ("VISA resource name out"=w343:refnum<visa-resource-name>, "error out"=w342:errorcluster)  [unwired: 9 in]
          }
          frame #1 {
            # "开始设置速度精度和绝对运动模式"
            n119 = VISA Write ("VISA写入")(VISA resource name=w355, write buffer="a\r" ("写入缓冲区"), error in (no error)=w354) -> (VISA resource name out=w362:refnum<visa-resource-name>, error out=w363:errorcluster)  [unwired: 1 out]
            n120 = VISA Read(VISA resource name=w362, byte count=u32 1 ("字节总数"), error in (no error)=w363) -> (VISA resource name out=w361:refnum<visa-resource-name>, error out=w360:errorcluster)  [unwired: 2 out]
            n121 = VISA Write ("VISA写入")(VISA resource name=w361, write buffer="Vô\u0001\r" ("写入缓冲区"), error in (no error)=w360) -> (VISA resource name out=w357:refnum<visa-resource-name>, error out=w358:errorcluster)  [unwired: 1 out]
            n122 = VISA Read(VISA resource name=w357, byte count=u32 1 ("字节总数"), error in (no error)=w358) -> (VISA resource name out=w353:refnum<visa-resource-name>, error out=w352:errorcluster)  [unwired: 2 out]
          }
          frame #2 {
            # "刷新输出坐标"
            n123 = VISA Write ("VISA写入")(VISA resource name=w372, write buffer="c\r" ("写入缓冲区"), error in (no error)=w371) -> (VISA resource name out=w376:refnum<visa-resource-name>, error out=w375:errorcluster)  [unwired: 1 out]
            n124 = flat-sequence {
              tunnel: [w383] -> w373
              tunnel: w376 -> [w383]
              tunnel: [w382] -> w374
              tunnel: w375 -> [w382]
              frame #0 {
                n125 = Wait (ms)(milliseconds to wait=u32 100 ("等待时间（毫秒）")) -> ()  [unwired: 1 out]
              }
            }
            n126 = property class="Instr"(reference=w373, error in=w374) -> (reference out=w378:refnum<visa-resource-name>, error out=w377:errorcluster, "Serial Settings:Number of Bytes at Serial Port"=w379:u32)
            n127 = VISA Read(VISA resource name=w378, byte count=w379, error in (no error)=w377) -> (VISA resource name out=w370:refnum<visa-resource-name>, read buffer=w381:string, error out=w369:errorcluster)  [unwired: 1 out]
            n128 = call "mp285_Move_str2xyz.vi"("字符串"=w381) -> ("X轴"=w368:dbl, "Y轴"=w367:dbl, "Z轴"=w366:dbl)
            n129 = local write "X."(w368) -> ()
            n130 = local write "Y."(w367) -> ()
            n131 = local write "Z."(w366) -> ()
          }
          frame #3 {
            # "刷新控制箱显示屏"
            n132 = VISA Write ("VISA写入")(VISA resource name=w388, write buffer="n\r" ("写入缓冲区"), error in (no error)=w387) -> (VISA resource name out=w391:refnum<visa-resource-name>, error out=w392:errorcluster)  [unwired: 1 out]
            n133 = VISA Read(VISA resource name=w391, byte count=u32 1 ("字节总数"), error in (no error)=w392) -> (VISA resource name out=w386:refnum<visa-resource-name>, error out=w385:errorcluster)  [unwired: 2 out]
          }
        }
      }
      event "设置当前位置为原点": Mouse Down {
        n134 = event-data() -> ()  [unwired: 1 in, 8 out]
        n135 = flat-sequence {
          tunnel: w401 -> [w406]
          tunnel: w400 -> [w405]
          tunnel: [w402] -> w399
          tunnel: [w404] -> w398
          tunnel: [w403] -> w397
          tunnel: w398 -> [w417]
          tunnel: w397 -> [w416]
          tunnel: [w415] -> w396
          tunnel: [w414] -> w395
          tunnel: w396 -> [w433]
          tunnel: w395 -> [w432]
          tunnel: [w431] -> w394
          tunnel: [w430] -> w393
          frame #0 {
            # "Set Origin"
            n136 = VISA Write ("VISA写入")(VISA resource name=w406, write buffer="o\r" ("写入缓冲区"), error in (no error)=w405) -> (VISA resource name out=w408:refnum<visa-resource-name>, error out=w407:errorcluster)  [unwired: 1 out]
            n137 = VISA Read(VISA resource name=w408, byte count=u32 1 ("字节总数"), error in (no error)=w407) -> (VISA resource name out=w404:refnum<visa-resource-name>, read buffer=w402:string, error out=w403:errorcluster)  [unwired: 1 out]
          }
          frame #1 {
            # "刷新输出坐标"
            n138 = VISA Write ("VISA写入")(VISA resource name=w417, write buffer="c\r" ("写入缓冲区"), error in (no error)=w416) -> (VISA resource name out=w421:refnum<visa-resource-name>, error out=w420:errorcluster)  [unwired: 1 out]
            n139 = flat-sequence {
              tunnel: [w428] -> w418
              tunnel: w421 -> [w428]
              tunnel: [w427] -> w419
              tunnel: w420 -> [w427]
              frame #0 {
                n140 = Wait (ms)(milliseconds to wait=u32 100 ("等待时间（毫秒）")) -> ()  [unwired: 1 out]
              }
            }
            n141 = property class="Instr"(reference=w418, error in=w419) -> (reference out=w423:refnum<visa-resource-name>, error out=w422:errorcluster, "Serial Settings:Number of Bytes at Serial Port"=w424:u32)
            n142 = VISA Read(VISA resource name=w423, byte count=w424, error in (no error)=w422) -> (VISA resource name out=w415:refnum<visa-resource-name>, read buffer=w426:string, error out=w414:errorcluster)  [unwired: 1 out]
            n143 = call "mp285_Move_str2xyz.vi"("字符串"=w426) -> ("X轴"=w413:dbl, "Y轴"=w412:dbl, "Z轴"=w411:dbl)
            n144 = local write "X."(w413) -> ()
            n145 = local write "Y."(w412) -> ()
            n146 = local write "Z."(w411) -> ()
          }
          frame #2 {
            # "刷新控制箱显示屏"
            n147 = VISA Write ("VISA写入")(VISA resource name=w433, write buffer="n\r" ("写入缓冲区"), error in (no error)=w432) -> (VISA resource name out=w436:refnum<visa-resource-name>, error out=w437:errorcluster)  [unwired: 1 out]
            n148 = VISA Read(VISA resource name=w436, byte count=u32 1 ("字节总数"), error in (no error)=w437) -> (VISA resource name out=w431:refnum<visa-resource-name>, error out=w430:errorcluster)  [unwired: 2 out]
          }
        }
      }
    }
    "字符串" <- w30
    n149 = local write "错误输出"(w28) -> ()
  }
  n150 = VISA Close(VISA resource name=w18, error in (no error)=w17) -> (error out=→"错误输出":errorcluster)
